vi "Corr2Coef U16.vi"(0 "Image A":u16[][](array[numeric]), 7 "Image B":u16[][](array[numeric]), 11 "Error In":errorcluster) -> (8 "Corr Coef":dbl, 15 "Error Out":errorcluster)   [LabVIEW 2020]
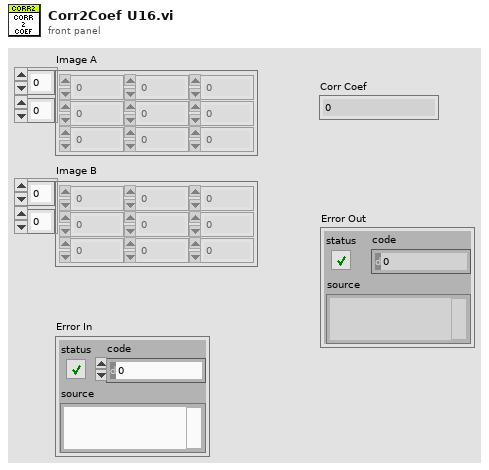
[diagram p1: front panel]
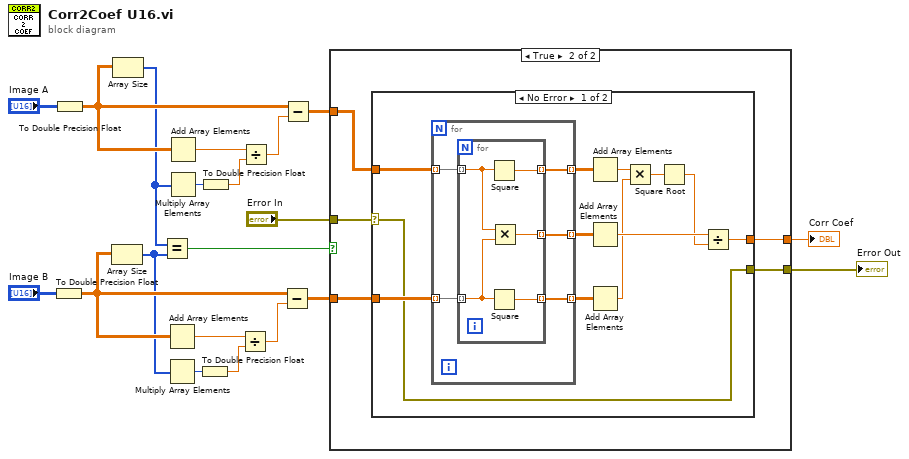
[diagram p0: block diagram]
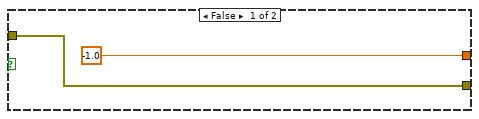
[diagram p2: hidden frame]
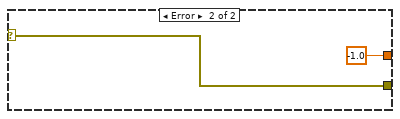
[diagram p3: hidden frame]
diagram:
  n1 = To Double Precision Float(number="Image B") -> (double precision float=w14:dbl[][])
  n2 = To Double Precision Float(number="Image A") -> (double precision float=w10:dbl[][])
  n3 = Array Size(array=w14) -> (size(s)=w4:i32[])
  n4 = Array Size(array=w10) -> (size(s)=w5:i32[])
  n5 = Equal?(x=w5, y=w4) -> (x = y?=w3:bool)
  n6 = Add Array Elements(numeric array=w14) -> (sum=w17:dbl)
  n7 = Multiply Array Elements(1:w4) -> (0:w16:i32)
  n8 = Add Array Elements(numeric array=w10) -> (sum=w7:dbl)
  n9 = Multiply Array Elements(1:w5) -> (0:w8:i32)
  n10 = To Double Precision Float(number=w16) -> (double precision float=w15:dbl)
  n11 = To Double Precision Float(number=w8) -> (double precision float=w9:dbl)
  n12 = Divide(x=w17, y=w15) -> (x/y=w13:dbl)
  n13 = Divide(x=w7, y=w9) -> (x/y=w11:dbl)
  n14 = Subtract(x=w14, y=w13) -> (x-y=w12:dbl[][])
  n15 = Subtract(x=w10, y=w11) -> (x-y=w2:dbl[][])
  n16 = case shown="True" w3 {
    tunnel: [-1.0 w27] -> w20
    tunnel: [w21 w26] -> w19
    tunnel: "Error In" -> [w21 w23]
    tunnel: w12 -> [_ w25]
    tunnel: w2 -> [_ w24]
    frame False {
    }
    frame True {
      n17 = case shown="No Error" w23 {
        selector: w23 -> [w28 w50]
        tunnel: [w31 -1.0] -> w27
        tunnel: w24 -> [w30 _]
        tunnel: w25 -> [w29 _]
        tunnel: [w28 w50] -> w26
        frame No Error {
          n18 = for {
            tunnel: w30 -> [w44] mode=indexing
            tunnel: w29 -> [w43] mode=indexing
            tunnel: [w42] -> w39 mode=indexing
            tunnel: [w41] -> w37 mode=indexing
            tunnel: [w40] -> w38 mode=indexing
            n19 = for {
              tunnel: w44 -> [w49] mode=indexing
              tunnel: w43 -> [w48] mode=indexing
              tunnel: [w47] -> w42 mode=indexing
              tunnel: [w46] -> w41 mode=indexing
              tunnel: [w45] -> w40 mode=indexing
              n20 = Square(x=w49) -> (x^2=w47:dbl)
              n21 = Square(x=w48) -> (x^2=w45:dbl)
              n22 = Multiply(x=w49, y=w48) -> (x*y=w46:dbl)
            }
          }
          n23 = Add Array Elements(numeric array=w39) -> (sum=w35:dbl)
          n24 = Add Array Elements(numeric array=w37) -> (sum=w36:dbl)
          n25 = Add Array Elements(numeric array=w38) -> (sum=w34:dbl)
          n26 = Multiply(x=w35, y=w34) -> (x*y=w33:dbl)
          n27 = Square Root(x=w33) -> (sqrt(x)=w32:dbl)
          n28 = Divide(x=w36, y=w32) -> (x/y=w31:dbl)
        }
        frame Error {
        }
      }
    }
  }
  "Corr Coef" <- w20
  "Error Out" <- w19
